vi "Find All Uses.Unique Control Ref.vi"(10 "controls":refnum<vi>[](array[refnum]), 11 "top cluster":refnum<vi>) -> (2 "selected control":refnum<vi>, 3 "unique?":bool)   [LabVIEW 2020]
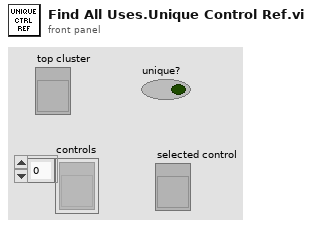
[diagram p1: front panel]
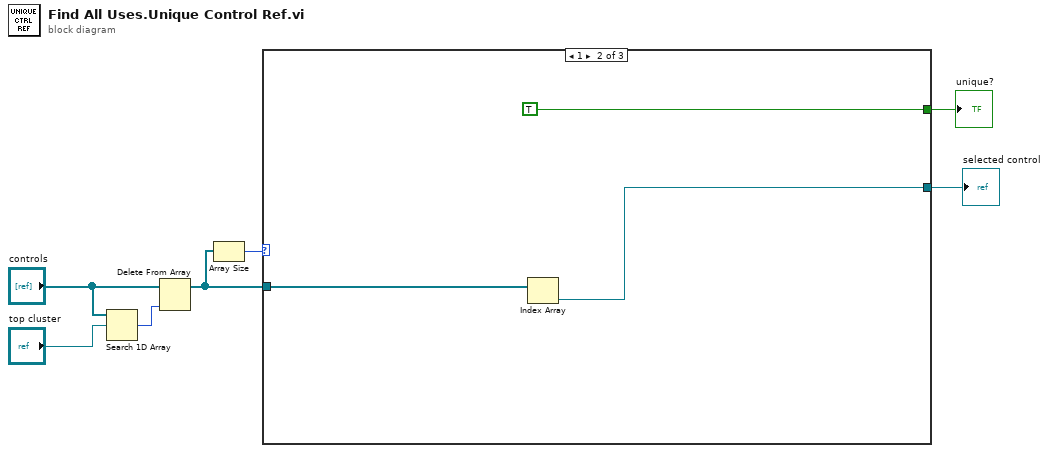
[diagram p0: block diagram]
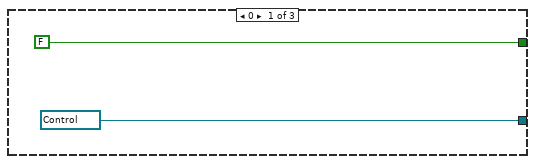
[diagram p2: hidden frame]
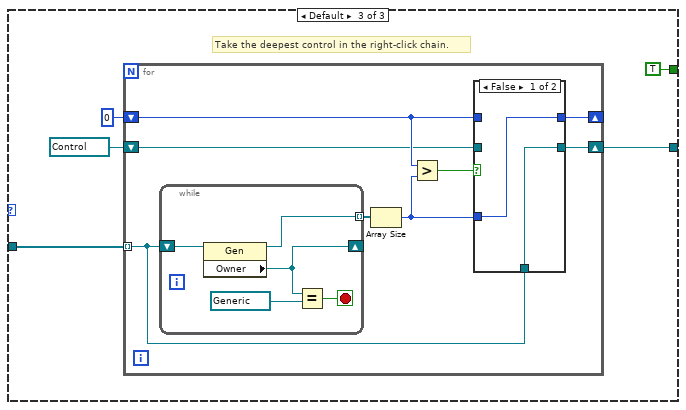
[diagram p3: hidden frame]
diagram:
  n1 = Search 1D Array(1D array="controls", element="top cluster") -> (index of element=w5:i32)  [unwired: 1 in]
  n2 = Delete From Array(array="controls", index=w5) -> (array with subset deleted=w2:refnum<vi>[])  [unwired: 1 in, 1 out]
  n3 = Array Size(array=w2) -> (size(s)=w4:i32)
  n4 = case shown="1" w4 {
    tunnel: [FALSE TRUE TRUE] -> w3
    tunnel: w2 -> [_ w11 w17]
    tunnel: [refnum<vi> refnum ("Ctl Refnum") w10 w13] -> w1
    frame 0 {
    }
    frame 1 {
      n5 = Index Array(array=w11) -> (element=w10:refnum<vi>)  [unwired: 1 in]
    }
    frame Default {
      # "Take the deepest control in the right-click chain."
      n6 = for {
        tunnel: w17 -> [w18] mode=indexing
        shift-right: [w23] -> _
        shift-left: 0 ("size(s)") -> [w22]
        shift-right: [w21] -> w13
        shift-left: refnum<vi> refnum ("Ctl Refnum") -> [w20]
        n7 = while {
          tunnel: [w33] -> w25 mode=indexing
          shift-right: [w31] -> _
          shift-left: w18 -> [w34]
          stop <- w30 stop-if-true
          n8 = property class="Gen"(reference=w34) -> (reference out=w33:refnum<vi>, "Owner"=w31:refnum<vi>)  [unwired: 1 in, 1 out]
          n9 = Equal?(x=w31, y=refnum<vi> refnum) -> (x = y?=w30:bool)
        }
        n10 = Array Size(array=w25) -> (size(s)=w19:i32)
        n11 = Greater?(x=w22, y=w19) -> (0:w24:bool)
        n12 = case shown="False" w24 {
          tunnel: [w27 w29] -> w23
          tunnel: w22 -> [_ w29]
          tunnel: [w26 w28] -> w21
          tunnel: w20 -> [_ w28]
          tunnel: w19 -> [w27 _]
          tunnel: w18 -> [w26 _]
          frame False {
          }
          frame True {
          }
        }
      }
    }
  }
  "selected control" <- w1
  "unique?" <- w3
